vi "藻密度单位换算.vi"(11 "藻密度显示":T1) -> (1 "数据标识":string, 2 "检测值1.单位":string, 3 "测量值":sgl)   [LabVIEW 2016, in "斯坦道多参数.lvlib"]
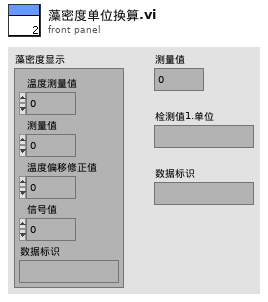
[diagram p1: front panel]
types:
  T1 = cluster{"温度测量值":sgl, "测量值":sgl, "温度偏移修正值":sgl, "信号值":sgl, "数据标识":string}
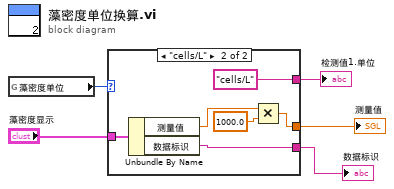
[diagram p0: block diagram]
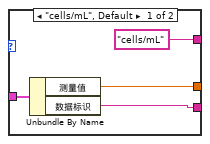
[diagram p2: hidden frame]
diagram:
  n1 = global read "断电保存变量.vi" "藻密度单位"() -> (w1:enum16{"cells/mL", "cells/L"})
  n2 = case shown="\"cells/L\"" w1 {
    tunnel: "藻密度显示" -> [w9 w15]
    tunnel: [w8 w11] -> w3
    tunnel: [w7 w13] -> w4
    tunnel: ["cells/mL" ("检测值1.单位") "cells/L" ("检测值1.单位")] -> w5
    frame "cells/mL", Default {
      n3 = Unbundle By Name(w9) -> ("测量值"=w8:sgl, "数据标识"=w7:string)
    }
    frame "cells/L" {
      n4 = Unbundle By Name(w15) -> ("测量值"=w14:sgl, "数据标识"=w13:string)
      n5 = Multiply(x=w14, y=sgl 1000.0) -> (x*y=w11:sgl)
    }
  }
  "检测值1.单位" <- w5
  "数据标识" <- w4
  "测量值" <- w3
